vi "CRYTree Navigate for Save.vi"(7 "Items":refnum<vi>, 9 "Type":enum16{"Curves", "Values", "Results", "WFM"}(ring), 10 "Start Tag In":string, 11 "Tree In":refnum<vi>) -> (3 "Tree Out":refnum<vi>)   [LabVIEW 2013]
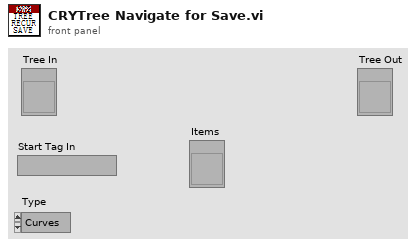
[diagram p1: front panel]
types:
  T1 = cluster{"Left Cell String":string, "Child Text":string[], "Child Tag":string, "Item Indent":i32, "Child Only?":bool, "Glyph Index":i32}[]
  T2 = cluster{"Left Cell String":string, "Child Text":string[], "Child Tag":string, "Item Indent":i32, "Child Only?":bool, "Glyph Index":i32}
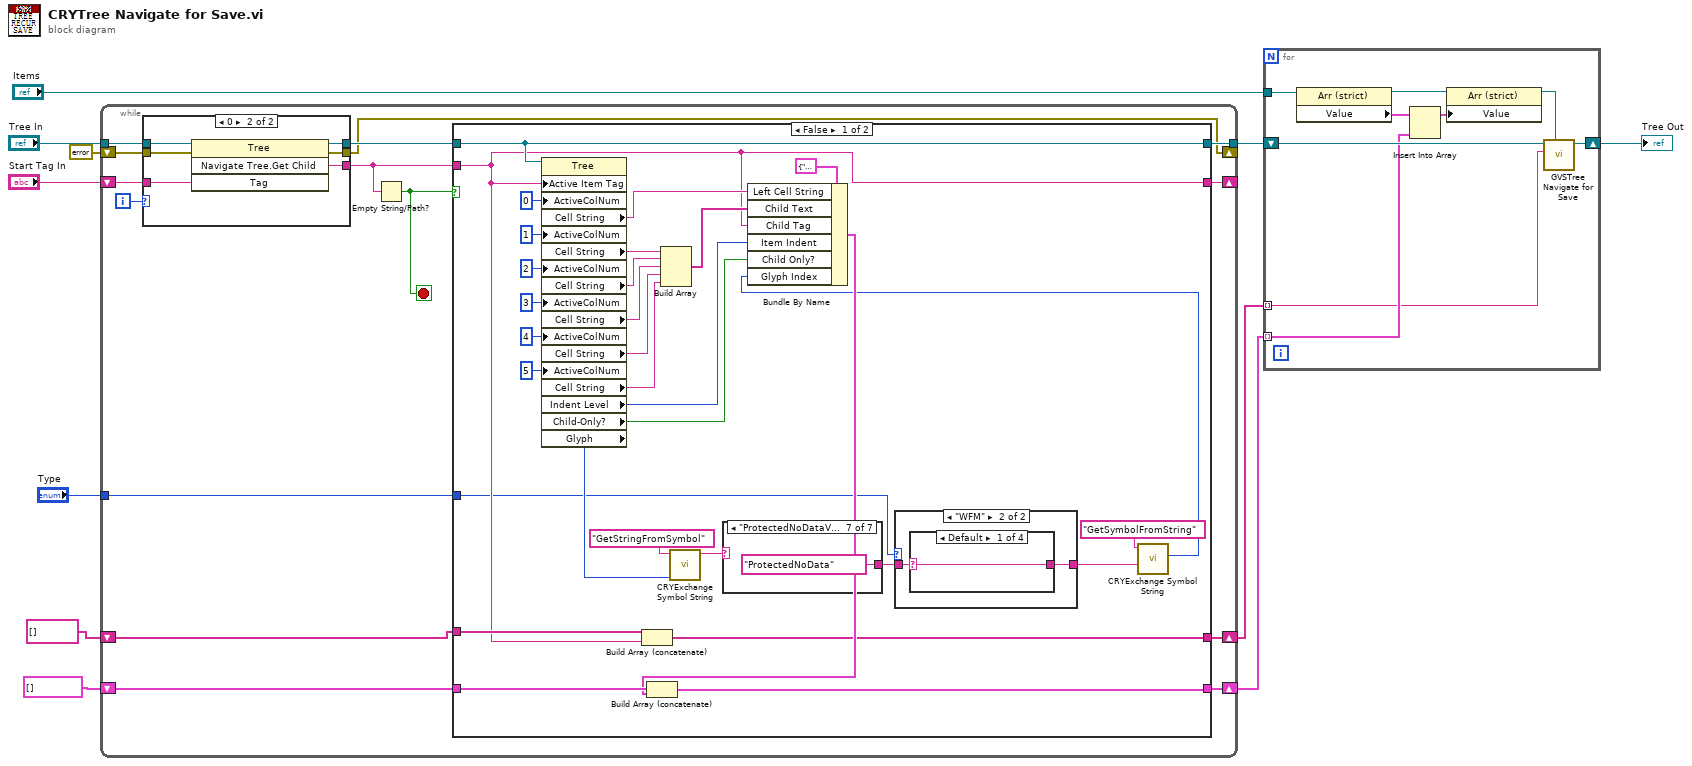
[diagram p0: block diagram]
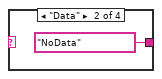
[diagram p3: hidden frame]
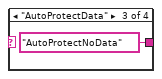
[diagram p4: hidden frame]
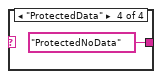
[diagram p5: hidden frame]
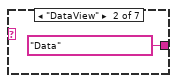
[diagram p7: hidden frame]
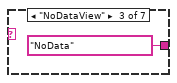
[diagram p8: hidden frame]
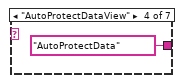
[diagram p9: hidden frame]
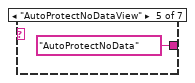
[diagram p10: hidden frame]
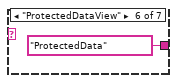
[diagram p11: hidden frame]
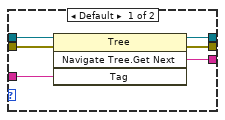
[diagram p13: hidden frame]
diagram:
  n1 = while {
    tunnel: "Tree In" -> [w26]
    shift-right: [w18] -> _
    shift-left: "Start Tag In" -> [w17]
    shift-right: [w15] -> _
    shift-left: errorcluster {"status"=FALSE, "code"=0, "source"=""} ("error out") -> [w24]
    shift-right: [w22] -> w2
    shift-left: T1 [] -> [w23]
    tunnel: [w20] -> w10
    shift-right: [w13] -> w3
    shift-left: string[] [] -> [w14]
    tunnel: "Type" -> [w12]
    i -> [w25]
    stop <- w16 stop-if-true
    n2 = case shown="0" w25 {
      tunnel: w26 -> [w81 w87]
      tunnel: w17 -> [w80 w86]
      tunnel: [w78 w85] -> w19
      tunnel: w24 -> [w79 w84]
      tunnel: [w77 w83] -> w15
      tunnel: [w76 w82] -> w21
      frame Default {
        n3 = invoke class="Tree" method="Navigate Tree.Get Next"(reference=w81, error in=w79, "Tag"=w80) -> (reference out=w76:refnum<vi>, error out=w77:errorcluster, "Navigate Tree:Get Next Item"=w78:string)  [unwired: 1 in, 1 out]
      }
      frame 0 {
        n4 = invoke class="Tree" method="Navigate Tree.Get Child"(reference=w87, error in=w84, "Tag"=w86) -> (reference out=w82:refnum<vi>, error out=w83:errorcluster, "Navigate Tree:Get Child"=w85:string)  [unwired: 1 in, 1 out]
      }
    }
    n5 = Empty String/Path?(string/path=w19) -> (empty?=w16:bool)
    n6 = case shown="False" w16 {
      tunnel: w23 -> [w57 w75]
      tunnel: [w56 w75] -> w22
      tunnel: w21 -> [w55 w73]
      tunnel: [w55 w73] -> w20
      tunnel: w19 -> [w35 w74]
      tunnel: [w35 w74] -> w18
      tunnel: w14 -> [w37 w72]
      tunnel: [w36 w72] -> w13
      tunnel: w12 -> [w29 _]
      frame False {
        n7 = property class="Tree"(reference=w55, "Active Item Tag"=w35, "ActiveColNum"=0 ("Active Cell:Active Column Number"), "ActiveColNum"=1 ("Active Cell:Active Column Number"), "ActiveColNum"=2 ("Active Cell:Active Column Number"), "ActiveColNum"=3 ("Active Cell:Active Column Number"), "ActiveColNum"=4 ("Active Cell:Active Column Number"), "ActiveColNum"=5 ("Active Cell:Active Column Number")) -> ("Cell String"=w52:string, "Cell String"=w46:string, "Cell String"=w45:string, "Cell String"=w44:string, "Cell String"=w43:string, "Cell String"=w42:string, "Indent Level"=w40:i32, "Child-Only?"=w39:bool, "Glyph"=w31:i32)  [unwired: 1 in, 2 out]
        n8 = Build Array (concatenate)(w37, w35) -> (w36:string[])
        n9 = Build Array(w46, w45, w44, w43, w42) -> (w41:string[])
        n10 = call "CRYExchange Symbol String.vi"("nData"=w31, "sAction"="GetStringFromSymbol") -> ("sData out"=w33:string)  [unwired: 8 in, 1 out]
        n11 = case shown="\"ProtectedNoDataView\"" w33 {
          selector: w33 -> [w65 _ _ _ _ _ _]
          tunnel: [w65 "Data" ("name or relative path") "NoData" ("name or relative path") "AutoProtectData" ("name or relative path") "AutoProtectNoData" ("name or relative path") "ProtectedData" ("name or relative path") "ProtectedNoData" ("name or relative path")] -> w28
          frame Default {
          }
          frame "DataView" {
          }
          frame "NoDataView" {
          }
          frame "AutoProtectDataView" {
          }
          frame "AutoProtectNoDataView" {
          }
          frame "ProtectedDataView" {
          }
          frame "ProtectedNoDataView" {
          }
        }
        n12 = case shown="\"WFM\"" w29 {
          tunnel: w28 -> [w58 w60]
          tunnel: [w58 w59] -> w27
          frame Default {
          }
          frame "WFM" {
            n13 = case shown="Default" w60 {
              selector: w60 -> [w61 _ _ _]
              tunnel: [w61 "NoData" ("name or relative path") "AutoProtectNoData" ("name or relative path") "ProtectedNoData" ("name or relative path")] -> w59
              frame Default {
              }
              frame "Data" {
              }
              frame "AutoProtectData" {
              }
              frame "ProtectedData" {
              }
            }
          }
        }
        n14 = call "CRYExchange Symbol String.vi"("sData"=w27, "sAction"="GetSymbolFromString") -> ("nData out"=w30:i32)  [unwired: 8 in, 1 out]
        n15 = Bundle By Name(cluster=T2 {"Left Cell String"="", "Child Text"=[], "Child Tag"="", "Item Indent"=0, "Child Only?"=FALSE, "Glyph Index"=0} ("Item"), "Left Cell String"=w52, "Child Text"=w41, "Child Tag"=w35, "Item Indent"=w40, "Child Only?"=w39, "Glyph Index"=w30) -> (w38:T2)
        n16 = Build Array (concatenate)(w57, w38) -> (w56:T1)
      }
      frame True {
      }
    }
  }
  n17 = for {
    tunnel: w2 -> [w95] mode=indexing
    tunnel: "Items" -> [w94]
    shift-right: [w89] -> w7
    shift-left: w10 -> [w96]
    tunnel: w3 -> [w88] mode=indexing
    n18 = property class="Arr (strict)"(reference=w94) -> (reference out=w93:refnum<vi>, "Value"=w90:T1)  [unwired: 1 in, 1 out]
    n19 = Insert Into Array(array=w90, new element=w95) -> (w92:T1)  [unwired: 1 in]
    n20 = property class="Arr (strict)"(reference=w93, "Value"=w92) -> (reference out=w91:refnum<vi>)  [unwired: 1 in, 1 out]
    n21 = call "GVSTree Navigate for Save.vi"("Items"=w91, "Start Tag In"=w88, "Tree In"=w96) -> ("Tree Out"=w89:refnum<vi>)  [unwired: 8 in]
  }
  "Tree Out" <- w7
